vi "Copy Library Item.vi"(8 "error in (no error)":errorcluster, 9 "Copy Name":string, 10 "Copy location":path, 11 "Library in":refnum<vi>) -> (0 "error out":errorcluster, 2 "New Lib Path":path, 3 "Library out":refnum<vi>)   [LabVIEW 2019, in "gRPC Scripting Tools.lvlib"]
uses:
  gRPC Scripting Tools.lvlib
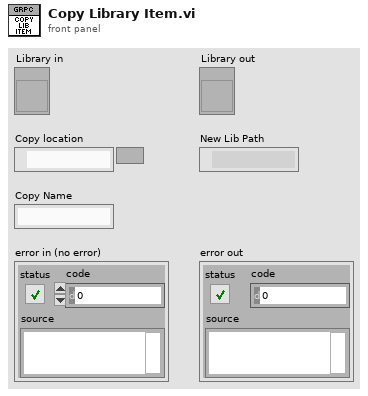
[diagram p1: front panel]
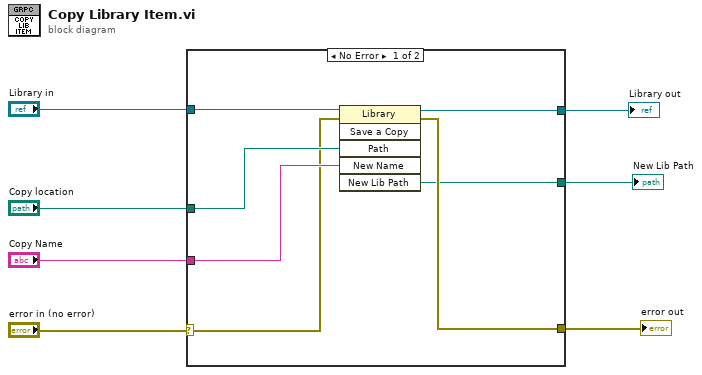
[diagram p0: block diagram]
diagram:
  n1 = case shown="No Error" "error in (no error)" {
    selector: "error in (no error)" -> [w8 w15]
    tunnel: [w14 w16] -> w7
    tunnel: [w13 w15] -> w6
    tunnel: "Library in" -> [w12 w16]
    tunnel: [w11 _] -> w4
    tunnel: "Copy Name" -> [w10 _]
    tunnel: "Copy location" -> [w9 _]
    frame No Error {
      n2 = invoke class="Library" method="Save a Copy"(reference=w12, error in=w8, "Path"=w9, "New Name"=w10) -> (reference out=w14:refnum<vi>, error out=w13:errorcluster, "New Lib Path"=w11:path)  [unwired: 2 in, 3 out]
    }
    frame Error {
    }
  }
  "Library out" <- w7
  "error out" <- w6
  "New Lib Path" <- w4
